vi "ResetDataLoopData.vi"() -> (3 "cluster":T1)   [LabVIEW 2016]
doc: "resets the data in the data loop clusterto default and/or empty values."
uses:
  DataLoopCluster.ctl
  SignalType.ctl
  range_cluster.ctl
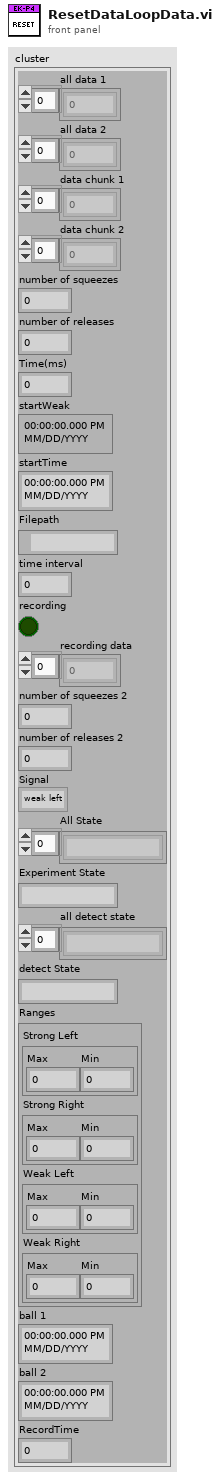
[diagram p1: front panel]
types:
  T1 = typedef "DataLoopCluster.ctl" = cluster{"all data 1":dbl[], "all data 2":dbl[], "data chunk 1":dbl[], "data chunk 2":dbl[], "number of squeezes":u16, "number of releases":u16, "Time(ms)":i64, "startWeak":timestamp, "startTime":timestamp, "Filepath":path, "time interval":u16, "recording":bool, "recording data":dbl[], "number of squeezes 2":u16, "number of releases 2":u16, "Signal":T2, "All State":string[], "Experiment State":string, "all detect state":string[], "detect State":string, "Ranges":cluster{"Strong Left":T3, "Strong Right":T3, "Weak Left":T3, "Weak Right":T3}, "ball 1":timestamp, "ball 2":timestamp, "RecordTime":u16}
  T2 = typedef "SignalType.ctl" = enum16{"weak left", "weak right", "strong left", "strong right"}
  T3 = typedef "range_cluster.ctl" = cluster{"Max":dbl, "Min":dbl}
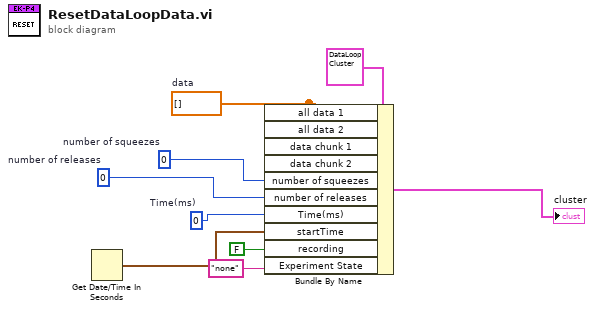
[diagram p0: block diagram]
diagram:
  w3 = i64 0  # Time(ms)
  w2 = u16 0  # number of releases
  w1 = u16 0  # number of squeezes
  w4 = dbl[] []  # data
  n1 = Get Date/Time In Seconds() -> (seconds since 1Jan1904=w7:timestamp)
  n2 = Bundle By Name(cluster=T1 {"all data 1"=[], "all data 2"=[], "data chunk 1"=[], "data chunk 2"=[], "number of squeezes"=0, "number of releases"=0, "Time(ms)"=0, "startWeak"=timestamp(0 s since 1904-01-01), "startTime"=timestamp(0 s since 1904-01-01), "Filepath"=path "", "time interval"=0, "recording"=FALSE, "recording data"=[], "number of squeezes 2"=0, "number of releases 2"=0, "Signal"=enum."weak left", "All State"=[], "Experiment State"="", "all detect state"=[], "detect State"="", "Ranges"={"Strong Left"={"Max"=0.0, "Min"=0.0}, "Strong Right"={"Max"=0.0, "Min"=0.0}, "Weak Left"={"Max"=0.0, "Min"=0.0}, "Weak Right"={"Max"=0.0, "Min"=0.0}}, "ball 1"=timestamp(0 s since 1904-01-01), "ball 2"=timestamp(0 s since 1904-01-01), "RecordTime"=0}, "all data 1"=w4, "all data 2"=w4, "data chunk 1"=w4, "data chunk 2"=w4, "number of squeezes"=w1, "number of releases"=w2, "Time(ms)"=w3, "startTime"=w7, "recording"=FALSE, "Experiment State"="none") -> (→"cluster":T1)
